vi "Start Command.vi"(8 "error in (no error)":errorcluster, 11 "Connect Command in":refnum<class "Connect Command.lvclass">) -> (0 "error out":errorcluster, 3 "Connect Command out":refnum<class "Connect Command.lvclass">)   [LabVIEW 2013, in "Receiver.lvlib" / "Receiver Commands Using Processor.lvlib" / "Connect Command.lvlib" / "Connect Command.lvclass"]
uses:
  Connect Command.lvclass
  Receiver Command.lvclass
  <vilib>/ActorFramework/Actor/Actor.lvclass/Actor.ctl
  <vilib>/ActorFramework/Message Enqueuer/Message Enqueuer.lvclass/Message Enqueuer.ctl
  <vilib>/ActorFramework/Message Enqueuer/Init from Existing Queue.vi
  <vilib>/ActorFramework/Message Enqueuer/Enqueue.vi
  <vilib>/ActorFramework/Message Priority Queue/Priority Enqueue.vi
  <vilib>/ActorFramework/Message Enqueuer/Message Enqueuer.lvclass
  Connect Command Messages/Go To Announcing Msg/Go To Announcing Msg.lvclass
  <vilib>/ActorFramework/Actor/Actor.lvclass
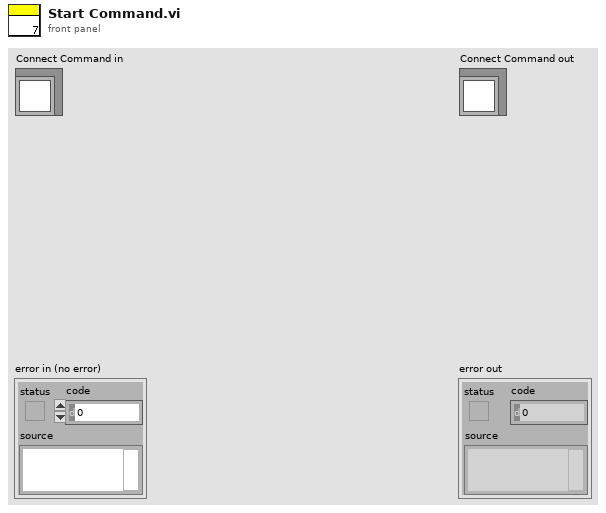
[diagram p1: front panel]
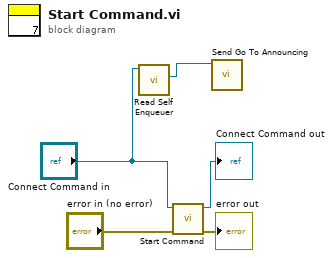
[diagram p0: block diagram]
diagram:
  n1 = call <vilib>:"Read Self Enqueuer.vi"("Actor"="Connect Command in") -> ("Self Enqueuer"=w1:refnum<class "Message Enqueuer.lvclass">)  [unwired: 10 in]
  n2 = call-parent "Start Command.vi"("error in (no error)"="error in (no error)", "Receiver Command in"="Connect Command in") -> ("error out"=→"error out":errorcluster, "Receiver Command out"=→"Connect Command out":refnum<class "Connect Command.lvclass">)  [unwired: 8 in]
  n3 = call "Send Go To Announcing.vi"("Message Enqueuer"=w1) -> ()  [unwired: 9 in, 2 out]
